vi "Straighten.vi"(8 "error in (no error)":errorcluster, 10 "Angle (rad)":dbl, 11 "Gantry In":refnum<k24>) -> (0 "error out":errorcluster, 3 "Gantry Out":refnum<k24>)   [LabVIEW 2020, in "A3200.lvclass"]
uses:
  A3200.lvclass
  Drivers/Aerotech A3200/Aerotech.lvlib
  Drivers/Aerotech A3200/Motion/MoveAbsSingle.vi
  C:/Program Files (x86)/Aerotech/A3200/LabVIEW/2010/Bin/Aerotech.A3200.dll
  Program Files (x86)/Aerotech/A3200/LabVIEW/2010/Bin/Aerotech.A3200.dll
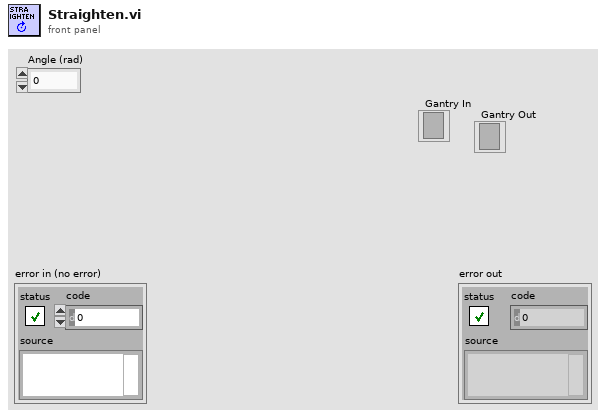
[diagram p1: front panel]
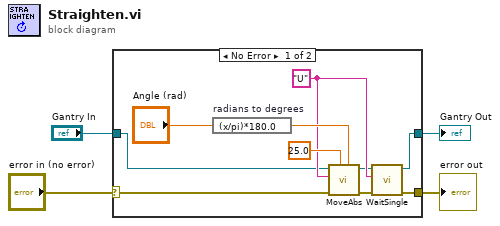
[diagram p0: block diagram]
diagram:
  n1 = case shown="No Error" "error in (no error)" {
    selector: "error in (no error)" -> [w7 w16]
    tunnel: [w5 w16] -> w3
    tunnel: "Gantry In" -> [w9 w15]
    tunnel: [w8 w15] -> w1
    frame No Error {
      w12 = "U" ("element")
      n2 = expression code="(x/pi)*180.0" "radians to degrees"("Angle (rad)") -> (w13:dbl)
      n3 = call-poly "MoveAbs.vi"("position"=w13, "speed"=25.0, "error in (no error)"=w7, "axis name"=w12, "controller in"=w9) -> ("error out"=w6:errorcluster, "controller out"=w11:refnum<k24>)  [unwired: 5 in]
      n4 = call "WaitSingle.vi"("error in (no error)"=w6, "axis name"=w12, "controller in"=w11) -> ("error out"=w5:errorcluster, "controller out"=w8:refnum<k24>)  [unwired: 6 in, 1 out]
    }
    frame Error {
    }
  }
  "error out" <- w3
  "Gantry Out" <- w1
